vi "APS get field bus last scan info.vi"(6 "Info_Count":i32, 7 "Array_Size":i32, 8 "error in (no error)":errorcluster caption="错误输入（无错误）", 9 "Info_Array":i32, 10 "BUS_No":i32, 11 "Board_ID":i32) -> (0 "error out":errorcluster caption="错误输出", 1 "Info_Array out":i32, 3 "function return":i32, 4 "Info_Count out":i32)   [LabVIEW 2011, in "APS168.lvlib"]
doc: "I32 FNTYPE APS_get_field_bus_last_scan_info( I32 Board_ID, I32 BUS_No, I32 *Info_Array, I32 Array_Size, I32 *Info_Count );"
uses:
  APS168.lvlib
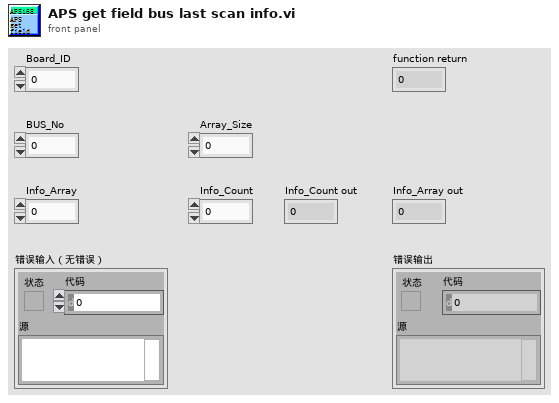
[diagram p1: front panel]
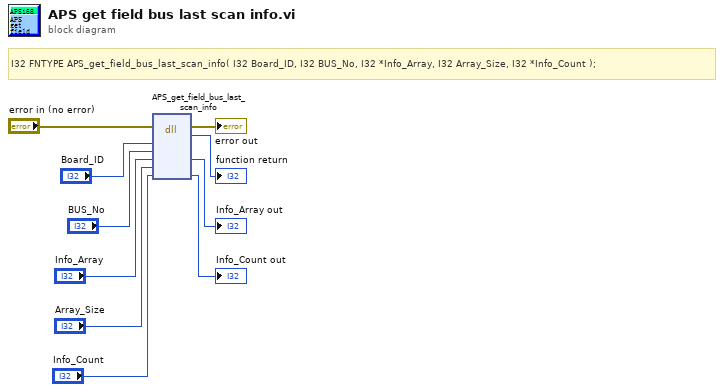
[diagram p0: block diagram]
diagram:
  # "I32 FNTYPE APS_get_field_bus_last_scan_info( I32 Board_ID, I32 BUS_No, I32 *Info_Array, I32 Array_Size, I32 *Info_Count );"
  n1 = dll-call lib="PTH1Labs E软件ADLINK 204CAPS_1_7_1_LIB line 连续运动204APS168.*" fn="APS_get_field_bus_last_scan_info"(error in="error in (no error)", "Board_ID"="Board_ID", "BUS_No"="BUS_No", "Info_Array"="Info_Array", "Array_Size"="Array_Size", "Info_Count"="Info_Count") -> (error out=→"error out":errorcluster, →"function return":i32, "Info_Array"=→"Info_Array out":i32, "Info_Count"=→"Info_Count out":i32)  [unwired: 5 in, 1 out]
